vi "Error Handler.vi"(7 "Dialog Title (\"\")":string, 8 "error in (no error)":errorcluster) -> (3 "Error?":bool)   [LabVIEW 2020, in "Output Sequencer.lvlib" / "Settings UI.lvclass"]
uses:
  Settings UI.lvclass
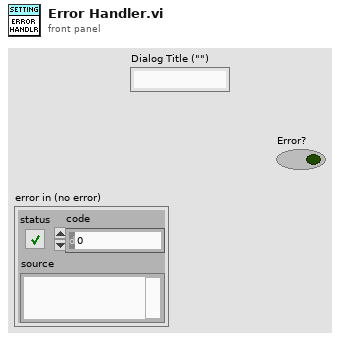
[diagram p1: front panel]
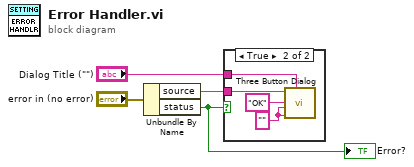
[diagram p0: block diagram]
diagram:
  n1 = Unbundle By Name("error in (no error)") -> ("source"=w2:string, "status"=w1:bool)
  "Error?" <- w1
  n2 = case shown="True" w1 {
    tunnel: w2 -> [_ w8]
    tunnel: "Dialog Title (\"\")" -> [_ w5]
    frame False {
    }
    frame True {
      w7 = "" ("Right Button Text (\"Cancel\")")
      n3 = call <vilib>:"Three Button Dialog.vi"("Window Title (\"\")"=w5, "Right Button Text (\"Cancel\")"=w7, "Center Button Text (\"No\")"=w7, "Left Button Text (\"Yes\")"="OK" ("Left Button Text (\"Yes\")"), "message"=w8) -> ()  [unwired: 6 in, 1 out]
    }
  }
